vi "BasHMIStart.vi"() -> ()   [LabVIEW 2019]
uses:
  <vilib>/Utility/sysdir.llb/System Directory Type.ctl
  <vilib>/NI/Current Value Table/DataTypes/Boolean_Write.vi
  <vilib>/NI/Current Value Table/Type to Enum.vi
  <vilib>/NI/Current Value Table/DataTypes/Boolean_Type To Enum.vi
  <vilib>/NI/Current Value Table/FGVs/CVT Globals.vi
  <vilib>/NI/Current Value Table/FGVs/Tag Memory.vi
  <vilib>/NI/Current Value Table/Memory Block.vi
  <vilib>/NI/Current Value Table/DataTypes/Boolean_Memory Block.vi
  <vilib>/NI/Current Value Table/Current Value Table.lvlib
panel:
  out "Loop Count":i32
  out "Stop":bool
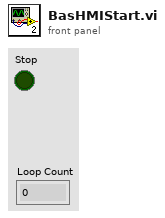
[diagram p1: front panel]
types:
  T1 = typedef "System Directory Type.ctl" = i32
  T2 = typedef "Current Value Table.lvlib/Single Tag.ctl" = cluster{"Data Type":T3, "Name":string, "Value":string, "Description":string}
  T3 = typedef "Current Value Table.lvlib/Data Types.ctl" = enum16{"Double", "Single", "I64", "I32", "I16", "I8", "U64", "U32", "U16", "U8", "String", "Boolean", "Array of U8", "Array of U16", "Array of U32", "Array of U64", "Array of I64", "Array of I32", "Array of I16", "Array of I8", "Array of Double", "Array of Single", "Array of Boolean", "Array of String"}
  T4 = typedef "tae_AlarmTagConfiguration.ctl" = cluster{"Name":string, "DataType":T5, "Alarm Configuration":T6}
  T5 = typedef "cvt_Data Types.ctl" = enum16{"Bool", "U8", "I32", "Double", "String", "Enum"}
  T6 = typedef "tae_AlarmConfiguration.ctl" = cluster{"Type":T7, "High Level":dbl, "Low Level":dbl, "Hysterisis":dbl, "Deadband":dbl}
  T7 = typedef "tae_AlarmType.ctl" = enum32{"Bool True", "Bool False", "Over Limit", "Under Limit", "Out-of-Range", "Enum Equal", "Enum Not Equal"}
  T8 = typedef "Current Value Table.lvlib/File Format.ctl" = cluster{"Tags":T2[], "Group Listings":T9[]}
  T9 = typedef "Current Value Table.lvlib/Tag Grouping set.ctl" = cluster{"Group":string, "Tag Names":string[]}
  T10 = typedef "tae_AlarmCommOut.ctl" = refnum<queue>
  T11 = typedef "tae_AlarmTagList.ctl" = T4[]
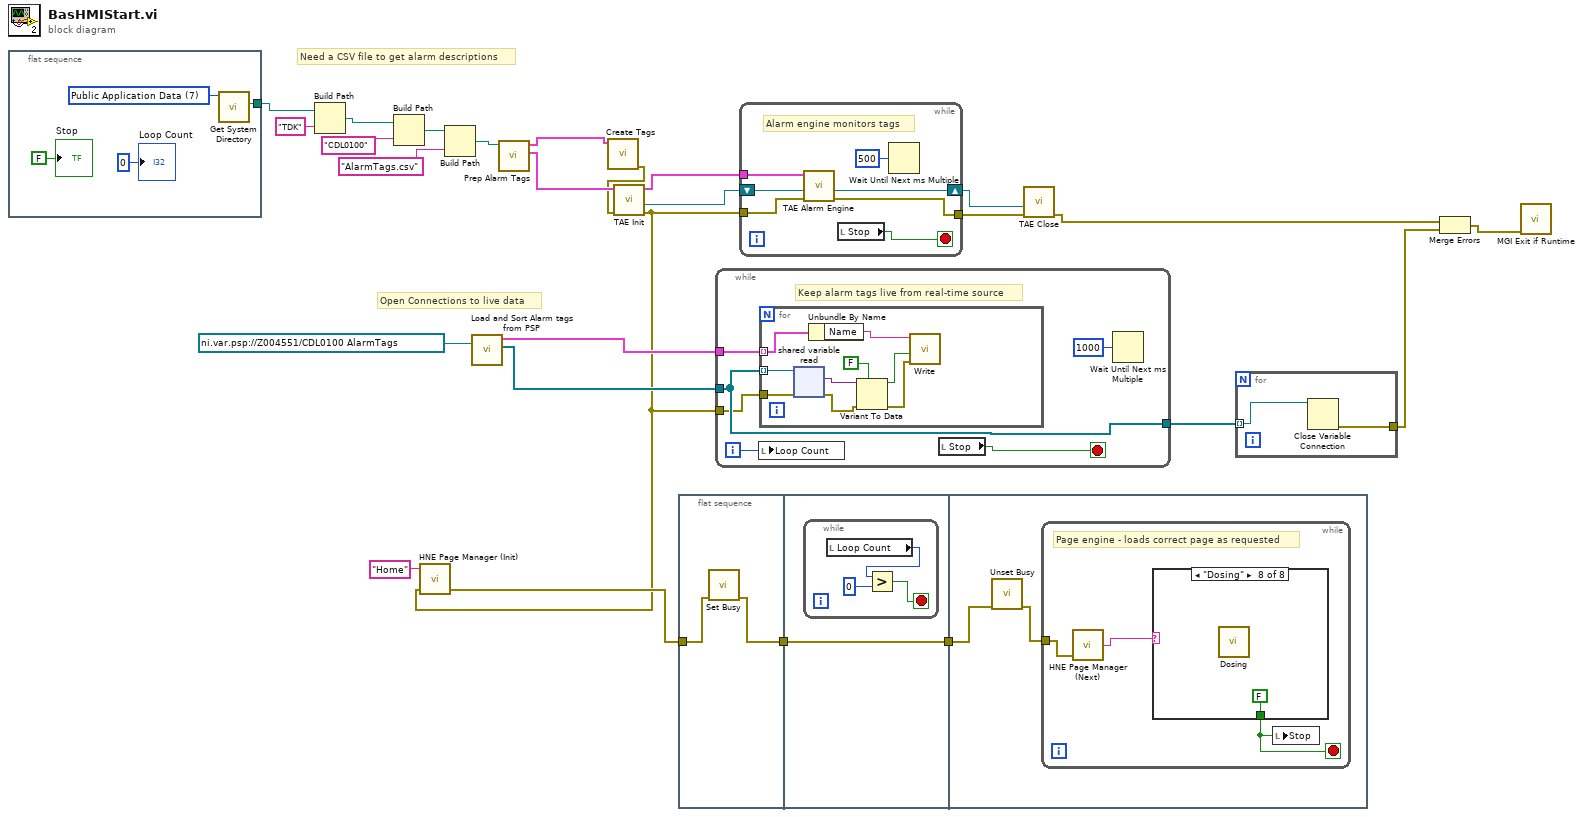
[diagram p0: block diagram]
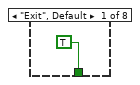
[diagram p2: hidden frame]
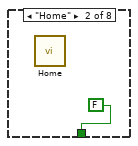
[diagram p3: hidden frame]
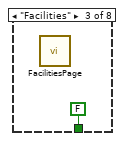
[diagram p4: hidden frame]
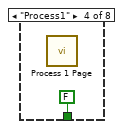
[diagram p5: hidden frame]
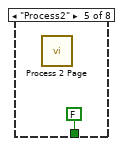
[diagram p6: hidden frame]
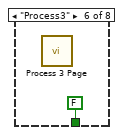
[diagram p7: hidden frame]
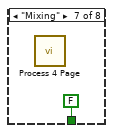
[diagram p8: hidden frame]
diagram:
  # "Open Connections to live data"
  # "Need a CSV file to get alarm descriptions"
  n1 = flat-sequence {
    tunnel: [w29] -> w25
    frame #0 {
      w30 = T1 7 items=["User Home"=0, "User Desktop"=1, "User Documents"=2, "User Application Data"=3, "User Preferences"=4, "User Temporary"=5, "Public Documents"=6, "Public Application Data"=7, "Public Preferences"=8, "Public Cache"=13, "System Core Libraries"=9, "System Installed Libraries"=10, "Application Files"=11, "Boot Volume Root"=12] ("system directory type")
      n2 = call <vilib>:"Get System Directory.vi"("system directory type"=w30) -> ("system directory"=w29:path)  [unwired: 10 in]
      "Loop Count" <- 0 ("Loop Count")
      "Stop" <- FALSE ("Stop")
    }
  }
  n3 = Build Path(base path=w25, name or relative path="TDK") -> (appended path=w23:path)
  n4 = Build Path(base path=w23, name or relative path="CDL0100") -> (appended path=w21:path)
  n5 = Build Path(base path=w21, name or relative path="AlarmTags.csv") -> (appended path=w19:path)
  n6 = call "Load and Sort Alarm tags from PSP.vi"("Refnum in"=refnum<k21> "ni.var.psp://Z004551/CDL0100 AlarmTags") -> ("Array 2"=w10:refnum<k21>[], "Array"=w9:T2[])  [unwired: 9 in]
  n7 = call "Prep Alarm Tags.vi"("Alarm Tag Description path"=w19) -> ("Alarm Array"=w17:T4[], "CVT Tags to Create"=w18:T8)  [unwired: 9 in]
  n8 = call <vilib>:"Create Tags.vi"("CVT Tags to Create"=w18) -> ("error out"=w6:errorcluster)  [unwired: 10 in]
  n9 = call <userlib>:"TAE Init.vi"("error in (no error)"=w6, "Alarm List"=w17) -> ("error out"=w7:errorcluster, "queue out"=w15:T10, "Alarm List"=w16:T11)  [unwired: 7 in]
  n10 = call <userlib>:"HNE Page Manager (Init).vi"("error in (no error)"=w7, "Initial Page"="Home") -> ("error out"=w11:errorcluster)  [unwired: 3 in]
  n11 = flat-sequence {
    tunnel: w11 -> [w32]
    tunnel: [w31] -> w4
    tunnel: [w33] -> w5
    tunnel: w4 -> [w33]
    tunnel: w5 -> [w38]
    frame #0 {
      n12 = call <vilib>:"Set Busy.vi"("error in (no error)"=w32) -> ("error out"=w31:errorcluster)  [unwired: 9 in, 1 out]
    }
    frame #1 {
      n13 = while {
        stop <- w36 stop-if-true
        n14 = local read "Loop Count"() -> (w35:i32)
        n15 = Greater?(x=w35, y=0) -> (0:w36:bool)
      }
    }
    frame #2 {
      n16 = call <vilib>:"Unset Busy.vi"("error in (no error)"=w38) -> ("error out"=w37:errorcluster)  [unwired: 10 in]
      n17 = while {
        tunnel: w37 -> [w39]
        stop <- w40 stop-if-true
        # "Page engine - loads correct page as requested"
        n18 = call <userlib>:"HNE Page Manager (Next).vi"("error in (no error)"=w39) -> ("Next Page"=w41:string)  [unwired: 3 in, 1 out]
        n19 = case shown="\"Dosing\"" w41 {
          tunnel: [TRUE FALSE FALSE FALSE FALSE FALSE FALSE FALSE] -> w40
          frame "Exit", Default {
          }
          frame "Home" {
            n20 = call "Home.vi"() -> ()  [unwired: 12 in]
          }
          frame "Facilities" {
            n21 = call "FacilitiesPage.vi"() -> ()  [unwired: 12 in]
          }
          frame "Process1" {
            n22 = call "Process 1 Page.vi"() -> ()  [unwired: 12 in]
          }
          frame "Process2" {
            n23 = call "Process 2 Page.vi"() -> ()  [unwired: 12 in]
          }
          frame "Process3" {
            n24 = call "Process 3 Page.vi"() -> ()  [unwired: 12 in]
          }
          frame "Mixing" {
            n25 = call "Process 4 Page.vi"() -> ()  [unwired: 12 in]
          }
          frame "Dosing" {
            n26 = call "Dosing.vi"() -> ()  [unwired: 12 in]
          }
        }
        n27 = local write "Stop"(w40) -> ()
      }
    }
  }
  n28 = while {
    tunnel: w10 -> [w53]
    tunnel: w9 -> [w55]
    tunnel: [w53] -> w8
    tunnel: w7 -> [w51]
    i -> [w50]
    stop <- w54 stop-if-true
    # "Keep alarm tags live from real-time source"
    n29 = local write "Loop Count"(w50) -> ()
    n30 = for {
      tunnel: w53 -> [w64] mode=indexing
      tunnel: w55 -> [w63] mode=indexing
      tunnel: w51 -> [w56]
      n31 = shared-variable-read(w64, w56) -> (w58:errorcluster, w61:variant)  [unwired: 2 out]
      n32 = Unbundle By Name(w63) -> ("Name"=w62:string)
      n33 = Variant To Data(error in=w58, type=FALSE, Variant=w61) -> (data=w59:bool, error out=w57:errorcluster)
      n34 = call-poly <vilib>:"Write.vi"("error in (no error)"=w57, "Value"=w59, "Tag Name"=w62) -> ()  [unwired: 8 in, 1 out]
    }
    n35 = local read "Stop"() -> (w54:bool)
    n36 = Wait Until Next ms Multiple(millisecond multiple=u32 1000) -> ()  [unwired: 1 out]
  }
  n37 = while {
    tunnel: w16 -> [w71]
    tunnel: w7 -> [w69]
    shift-right: [w68] -> w14
    shift-left: w15 -> [w70]
    tunnel: [w66] -> w13
    stop <- w65 stop-if-true
    # "Alarm engine monitors tags"
    n38 = call <userlib>:"TAE Alarm Engine.vi"("error out"=w69, "AE_CommIn"=w70, "Alarm List"=w71) -> ("error out 2"=w66:errorcluster, "Alarm queue out"=w68:T10)  [unwired: 6 in, 1 out]
    n39 = local read "Stop"() -> (w65:bool)
    n40 = Wait Until Next ms Multiple(millisecond multiple=u32 500) -> ()  [unwired: 1 out]
  }
  n41 = call <userlib>:"TAE Close.vi"("error in"=w13, "Alarm queue out"=w14) -> ("error out"=w3:errorcluster)  [unwired: 9 in]
  n42 = for {
    tunnel: w8 -> [w73] mode=indexing
    tunnel: [w72] -> w2
    n43 = Close Variable Connection(11:w73) -> (0:w72:errorcluster)  [unwired: 1 in]
  }
  n44 = Merge Errors(w3, w2) -> (w1:errorcluster)
  n45 = call <userlib>:"MGI Exit if Runtime.vi"("Error In (Dependency Only)"=w1) -> ()  [unwired: 11 in]
